vi "Speed_Selection(SSM).vi"(1 "SPEED(1~4)":string, 3 "baud rate (9600)":u32=115200 caption="보 전송속도(9600)", 4 "AXIS":u16(ring) items=["X", "Y"], 5 "Port":refnum<visa-resource-name>="COM4" caption="VISA 리소스 이름") -> (0 "Error Out":errorcluster caption="에러 출력", 2 "VISA out":refnum<visa-resource-name>)   [LabVIEW 2016]
uses:
  <vilib>/Instr/_visa.llb/VISA Configure Serial Port (Instr).vi
  <vilib>/Instr/_visa.llb/VISA Flush IO Buffer Mask.ctl
panel:
  out "Commend Count":u32
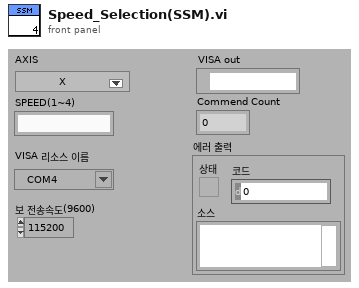
[diagram p1: front panel]
types:
  T1 = typedef "VISA Flush IO Buffer Mask.ctl" = u16
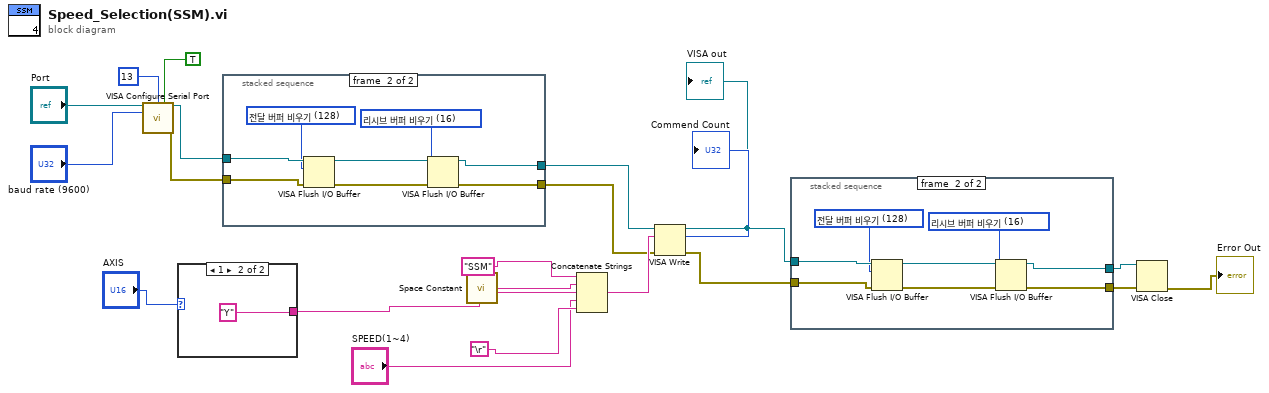
[diagram p0: block diagram]
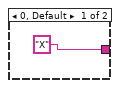
[diagram p2: hidden frame]
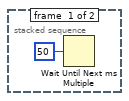
[diagram p3: hidden frame]
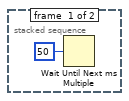
[diagram p4: hidden frame]
diagram:
  n1 = call-poly "VISA Configure Serial Port"("VISA resource name"="Port", "termination char\n(0xA = '\\n' = LF)"=i16 13 ("termination char\n(0xA = '\\n' = LF)"), "Enable Termination\nChar (T)"=TRUE ("Enable Termination\nChar (T)"), "baud rate (9600)"="baud rate (9600)") -> ("VISA resource name out"=w11:refnum<visa-resource-name>, "error out"=w10:errorcluster)  [unwired: 10 in]
  n2 = case shown="1" "AXIS" {
    tunnel: ["X" "Y"] -> w1
    frame 0, Default {
    }
    frame 1 {
    }
  }
  n3 = stacked-sequence {
    tunnel: w11 -> [_ w32]
    tunnel: w10 -> [_ w31]
    tunnel: [_ w27] -> w4
    tunnel: [_ w26] -> w3
    frame #0 {
      n4 = Wait Until Next ms Multiple(millisecond multiple=u32 50 ("ms 배수")) -> ()  [unwired: 1 out]
    }
    frame #1 {
      w25 = T1 16 items=["리시브 버퍼 비우기"=16, "전달 버퍼 디바이스에 쓰기"=32, "리시브 버퍼 비우기(I/O 없음)"=64, "전달 버퍼 비우기"=128] ("Mask")
      w30 = T1 128 items=["리시브 버퍼 비우기"=16, "전달 버퍼 디바이스에 쓰기"=32, "리시브 버퍼 비우기(I/O 없음)"=64, "전달 버퍼 비우기"=128] ("Mask")
      n5 = VISA Flush I/O Buffer(VISA resource name=w32, mask (16)=w30, error in (no error)=w31) -> (VISA resource name out=w29:refnum<visa-resource-name>, error out=w28:errorcluster)
      n6 = VISA Flush I/O Buffer(VISA resource name=w29, mask (16)=w25, error in (no error)=w28) -> (VISA resource name out=w27:refnum<visa-resource-name>, error out=w26:errorcluster)
    }
  }
  n7 = call <vilib>:"Space Constant.vi"() -> ("String"=w20:string)
  n8 = Concatenate Strings("SSM", w20, w1, "SPEED(1~4)", "\r") -> (w19:string)
  n9 = VISA Write(VISA resource name=w4, write buffer=w19, error in (no error)=w3) -> (VISA resource name out=w6:refnum<visa-resource-name>, return count=→"Commend Count":u32, error out=w5:errorcluster)
  "VISA out" <- w6
  n10 = stacked-sequence {
    tunnel: w6 -> [_ w41]
    tunnel: w5 -> [_ w40]
    tunnel: [_ w36] -> w8
    tunnel: [_ w35] -> w9
    frame #0 {
      n11 = Wait Until Next ms Multiple(millisecond multiple=u32 50 ("ms 배수")) -> ()  [unwired: 1 out]
    }
    frame #1 {
      w34 = T1 16 items=["리시브 버퍼 비우기"=16, "전달 버퍼 디바이스에 쓰기"=32, "리시브 버퍼 비우기(I/O 없음)"=64, "전달 버퍼 비우기"=128] ("Mask")
      w39 = T1 128 items=["리시브 버퍼 비우기"=16, "전달 버퍼 디바이스에 쓰기"=32, "리시브 버퍼 비우기(I/O 없음)"=64, "전달 버퍼 비우기"=128] ("Mask")
      n12 = VISA Flush I/O Buffer(VISA resource name=w41, mask (16)=w39, error in (no error)=w40) -> (VISA resource name out=w38:refnum<visa-resource-name>, error out=w37:errorcluster)
      n13 = VISA Flush I/O Buffer(VISA resource name=w38, mask (16)=w34, error in (no error)=w37) -> (VISA resource name out=w36:refnum<visa-resource-name>, error out=w35:errorcluster)
    }
  }
  n14 = VISA Close(VISA resource name=w8, error in (no error)=w9) -> (error out=→"Error Out":errorcluster)
